vi "Scaler_Rate.vi"() -> ()   [LabVIEW 2014]
panel:
  out "error out":errorcluster
  in  "error in (no error)":errorcluster
  in  "notifier":refnum<notifier>
  in  "Delay Time (s)":sgl=1.0
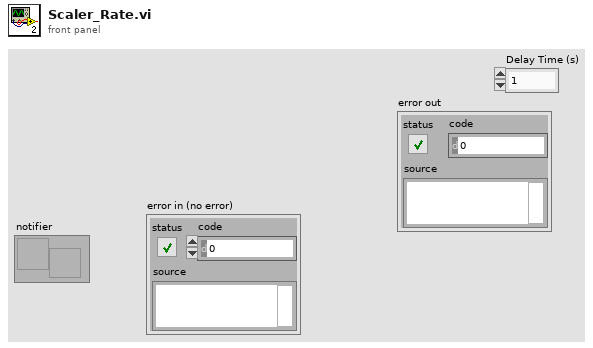
[diagram p1: front panel]
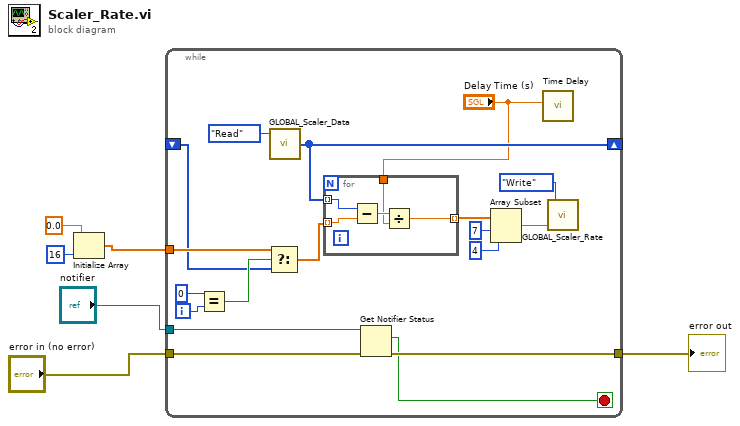
[diagram p0: block diagram]
diagram:
  n1 = Initialize Array(0.0 ("element"), 16 ("dimension size")) -> (w4:dbl[])
  n2 = while {
    shift-right: [w23] -> _
    shift-left: _ -> [w17]
    tunnel: w4 -> [w18]
    tunnel: "notifier" -> [w12]
    tunnel: "error in (no error)" -> [w11]
    tunnel: [w10] -> w1
    i -> [w21]
    stop <- w9 stop-if-true
    n3 = Equal?(x=0, y=w21) -> (x = y?=w19:bool)
    n4 = Select(t=w18, s=w19, f=w17) -> (s? t:f=w16:dbl[])
    n5 = call "GLOBAL_Scaler_Data.vi"("State"=enum16{"Initialise", "Write", "Read"}."Read") -> ("Data Out"=w23:u32[])  [unwired: 4 in]
    n6 = for {
      tunnel: w23 -> [w29] mode=indexing
      tunnel: w16 -> [w28] mode=indexing
      tunnel: "Delay Time (s)" -> [w26]
      tunnel: [w25] -> w15 mode=indexing
      n7 = Subtract(x=w29, y=w28) -> (x-y=w27:dbl)
      n8 = Divide(x=w27, y=w26) -> (x/y=w25:dbl)
    }
    n9 = Get Notifier Status(notifier=w12, error in (no error)=w11) -> (current notification=w9:bool, error out=w10:errorcluster)  [unwired: 3 out]
    n10 = Array Subset(array=w15, index=7, length=4) -> (w8:dbl[])
    n11 = call "Time Delay"("Delay Time (s)"="Delay Time (s)") -> ()  [unwired: 10 in, 1 out]
    n12 = call "GLOBAL_Scaler_Rate.vi"("Data in"=w8, "State"=enum16{"Initialise", "Write", "Read"}."Write") -> ()  [unwired: 3 in, 1 out]
  }
  "error out" <- w1
